vi "To Integer Tree Data.vi"(10 "Integer":i64) -> (3 "Integer Tree Data":refnum<class "Int.lvclass">)   [LabVIEW 2020, in "NI_VIAnCFGDataStructure.lvlib" / "Int.lvclass"]
doc: "Convert an Integer value to Tree Data type."
uses:
  <vilib>/addons/analyzer/VIAnCFGDataStructure/Data Types/Int/Int.lvclass
  <vilib>/addons/analyzer/VIAnCFGDataStructure/Data Types/Int/Int.lvclass/Int.ctl
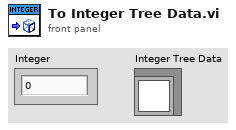
[diagram p1: front panel]
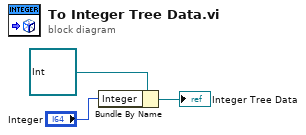
[diagram p0: block diagram]
diagram:
  n1 = Bundle By Name(cluster=refnum<class "Int.lvclass"> refnum ("Int in"), "Integer"="Integer") -> (→"Integer Tree Data":refnum<class "Int.lvclass">)
